vi "AH2700_Open_Queue.vi"(8 "error in (no error)":errorcluster caption="Fehler (Eingang, kein Fehler)") -> (0 "error out":errorcluster caption="Fehler (Ausgang)", 2 "queue out":refnum<queue>)   [LabVIEW 2019]
uses:
  AH2700/AH2700-Control.ctl
  Global/Global Variables/Queues_global.vi
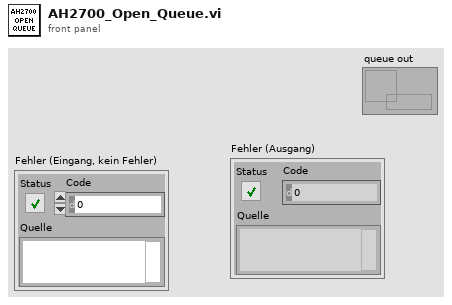
[diagram p1: front panel]
types:
  T1 = typedef "AH2700-Control.ctl" = cluster{"Update AH2500":bool}
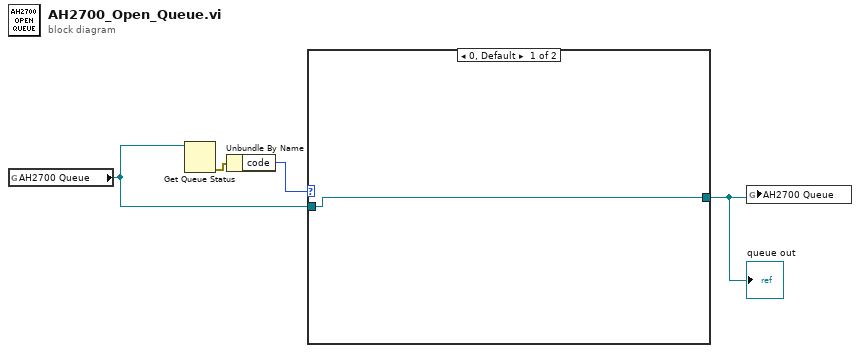
[diagram p0: block diagram]
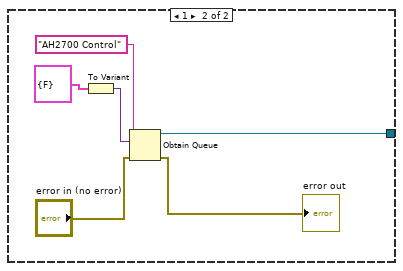
[diagram p2: hidden frame]
diagram:
  n1 = global read "Queues_global.vi" "AH2700 Queue"() -> (w2:refnum<queue>)
  n2 = Get Queue Status(queue=w2) -> (error out=w4:errorcluster)  [unwired: 2 in, 7 out]
  n3 = Unbundle By Name(w4) -> ("code"=w3:i32)
  n4 = case shown="0, Default" w3 {
    tunnel: w2 -> [w5 _]
    tunnel: [w5 w6] -> w1
    frame 0, Default {
    }
    frame 1 {
      n5 = To Variant(anything=T1 {"Update AH2500"=FALSE} ("AH2700-Control")) -> (Variant=w10:variant)
      n6 = Obtain Queue(name (unnamed)="AH2700 Control", element data type=w10, error in (no error)="error in (no error)") -> (queue out=w6:refnum<queue>, error out=→"error out":errorcluster)  [unwired: 2 in, 1 out]
    }
  }
  "queue out" <- w1
  n7 = global write "Queues_global.vi" "AH2700 Queue"(w1) -> ()
